vi "Data_filtering_test.vi"() -> ()   [LabVIEW 2018]
uses:
  <vilib>/Analysis/NI_AALBase.lvlib
  Tracker.lvlib
  <vilib>/Analysis/NI_AALPro.lvlib
  <vilib>/Analysis/baseanly.llb/Mean (DBL).vi
  SubVi's/Controls/CTL_Filter_selector.ctl
panel:
  out "X MSE, filt end HB":dbl format="%0.2f"
  out "Mean, coords HB + speed SG d1":dbl format="%0.2f"
  out "Speed MSE, coords HB + speed SG d1":dbl format="%0.2f"
  in  "HB filter length":i32=31
  out "Mean, coords SG + speed SG d1":dbl format="%0.2f"
  out "Mean, speed SG d1":dbl format="%0.2f"
  out "Mean, coords SG + speed HB":dbl format="%0.2f"
  out "Mean ideal speed":dbl format="%0.2f"
  out "Speed MSE, coords SG + speed HB":dbl format="%0.2f"
  out "Speed MSE, speed SG d1":dbl format="%0.2f"
  out "Speed MSE, coords SG + speed SG d1":dbl format="%0.2f"
  in  "Noise SD":dbl=3.0 min=0.0 max=10.0 step=0.1 format="%#_13g"
  out "Y MSE, filt on raw":dbl format="%0.2f"
  out "Y MSE, filt on end":dbl format="%0.2f"
  out "X MSE, filt on end":dbl format="%0.2f"
  out "X MSE, filt on raw":dbl format="%0.2f"
  out "Speed data":dbl[][](graph)
  in  "Filter parameters 2":T1={"Filter type"=enum."Savitzky-Golay", "Length"=31, "Order"=3} {"Order" min=3 max=11 step=2; "Length" min=5 max=301 step=2}
  out "Proc data":dbl[][](graph)
  in  "Filter parameters":T1={"Filter type"=enum."Savitzky-Golay", "Length"=31, "Order"=3} {"Order" min=3 max=11 step=2; "Length" min=5 max=301 step=2}
  out "Noisy raw data":dbl[][](graph)
  out "Pure raw data":dbl[][](graph)
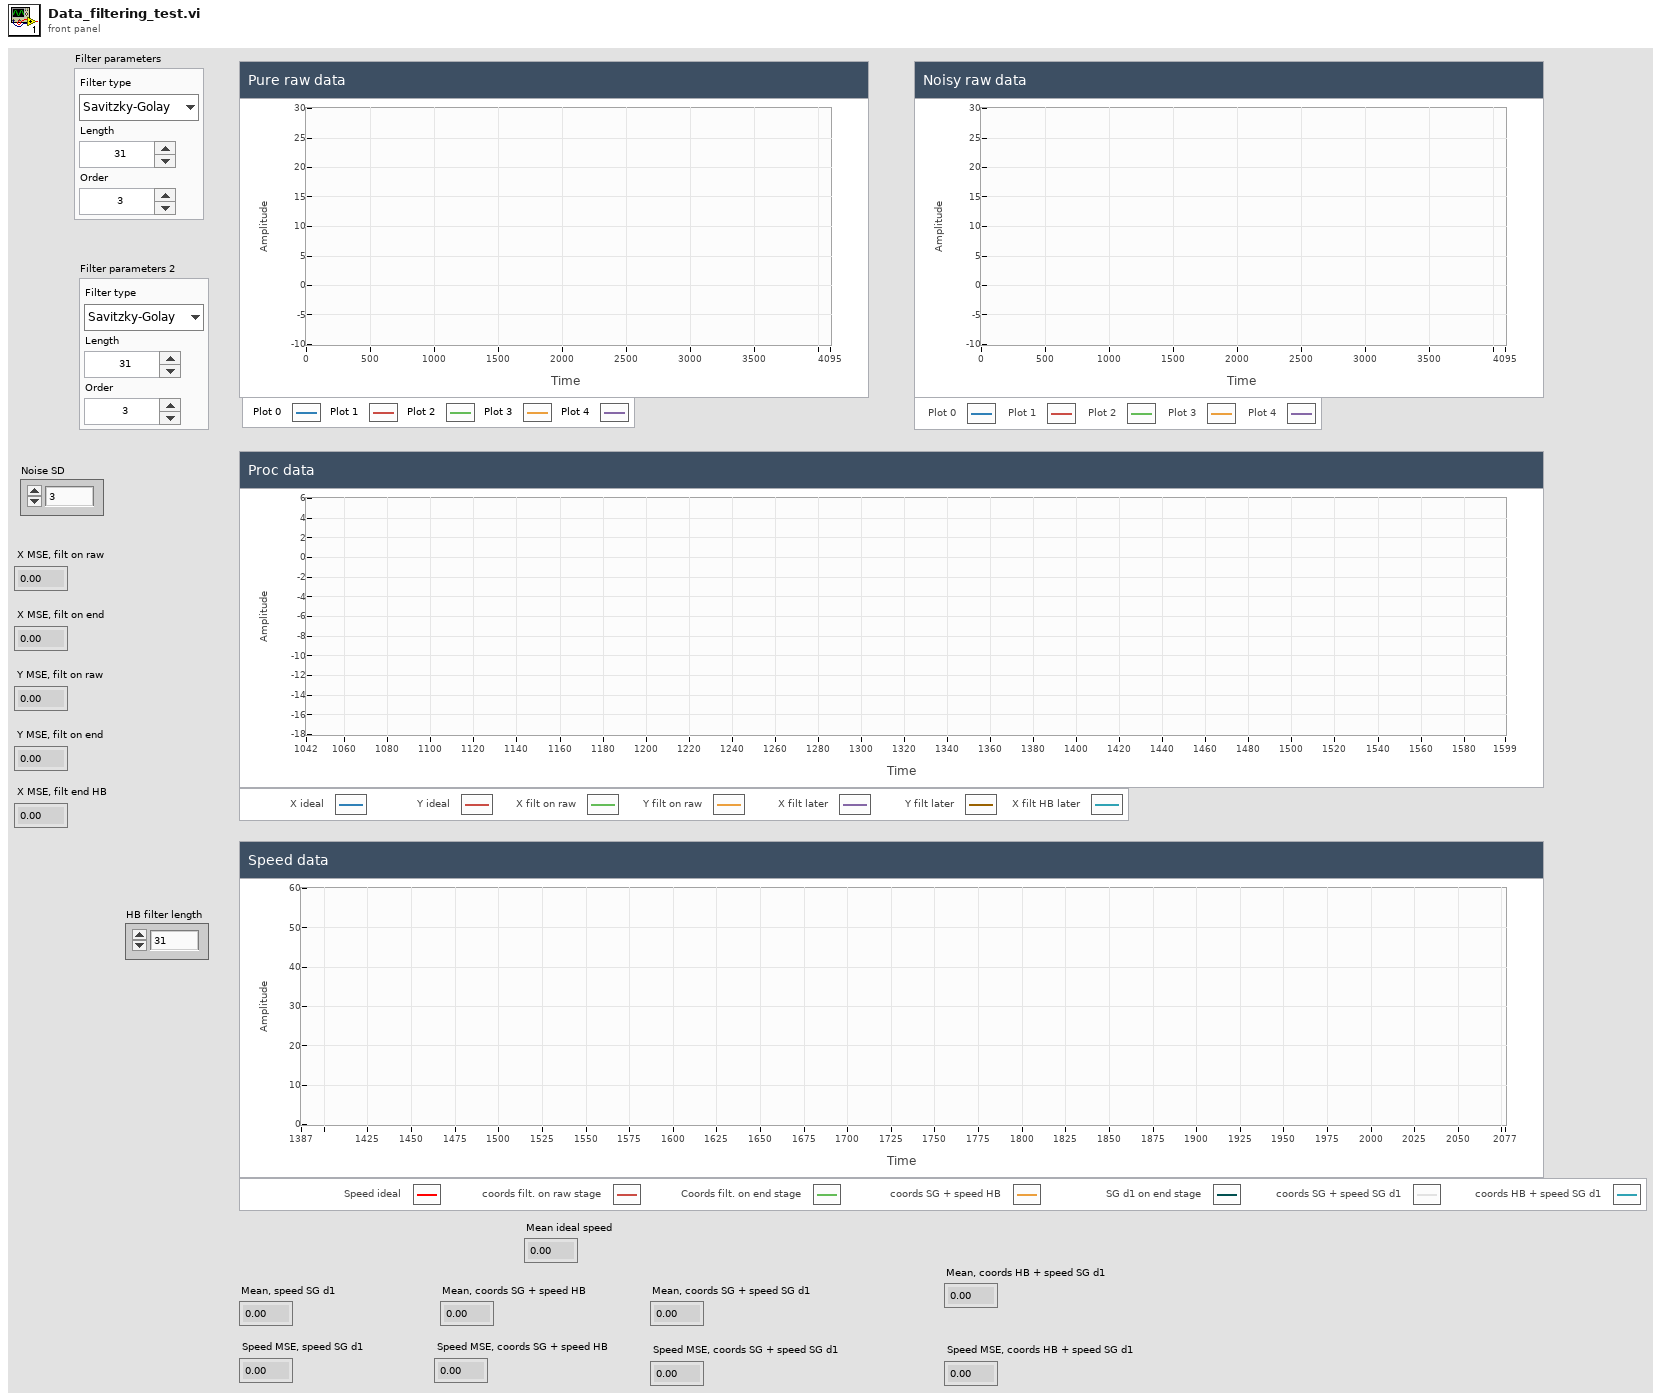
[diagram p1: front panel]
types:
  T1 = typedef "Tracker.lvlib/CTL_Filter_selector.ctl" = cluster{"Filter type":enum16{"None", "Savitzky-Golay"}, "Length":i32, "Order":i32}
  T2 = cluster{"ms since ON":u32, "delta time":u32, "X1":sgl, "Y1":sgl, "X2":sgl, "Y2":sgl, "TTL in 1":i16, "TTL in 2":i16, "Frame timestamp":timestamp, "Frame OK":bool}
  T3 = cluster{"X1 raw":dbl, "Y1 raw":dbl, "X2 raw":dbl, "Y2 raw":dbl}
  T4 = typedef "Tracker.lvlib/CTL_Cage_Coords.ctl" = cluster{"R from center":dbl, "sin(a)":dbl, "Mouse Xc":dbl, "Mouse Yc":dbl, "X1-X2":dbl, "Y1-Y2":dbl, "Cage Xc":dbl, "Cage Yc":dbl, "Frame time, s":dbl}
  T5 = cluster{"R from center":dbl, "phi (mouse angular position in the cage)":dbl, "alpha (mouse rot. angle)":sgl, "X":dbl, "Y":dbl, "theta (from center towards mouse)":dbl, "beta (cage rot. against mouse)":sgl, "w (mouse angle to wall)":dbl}
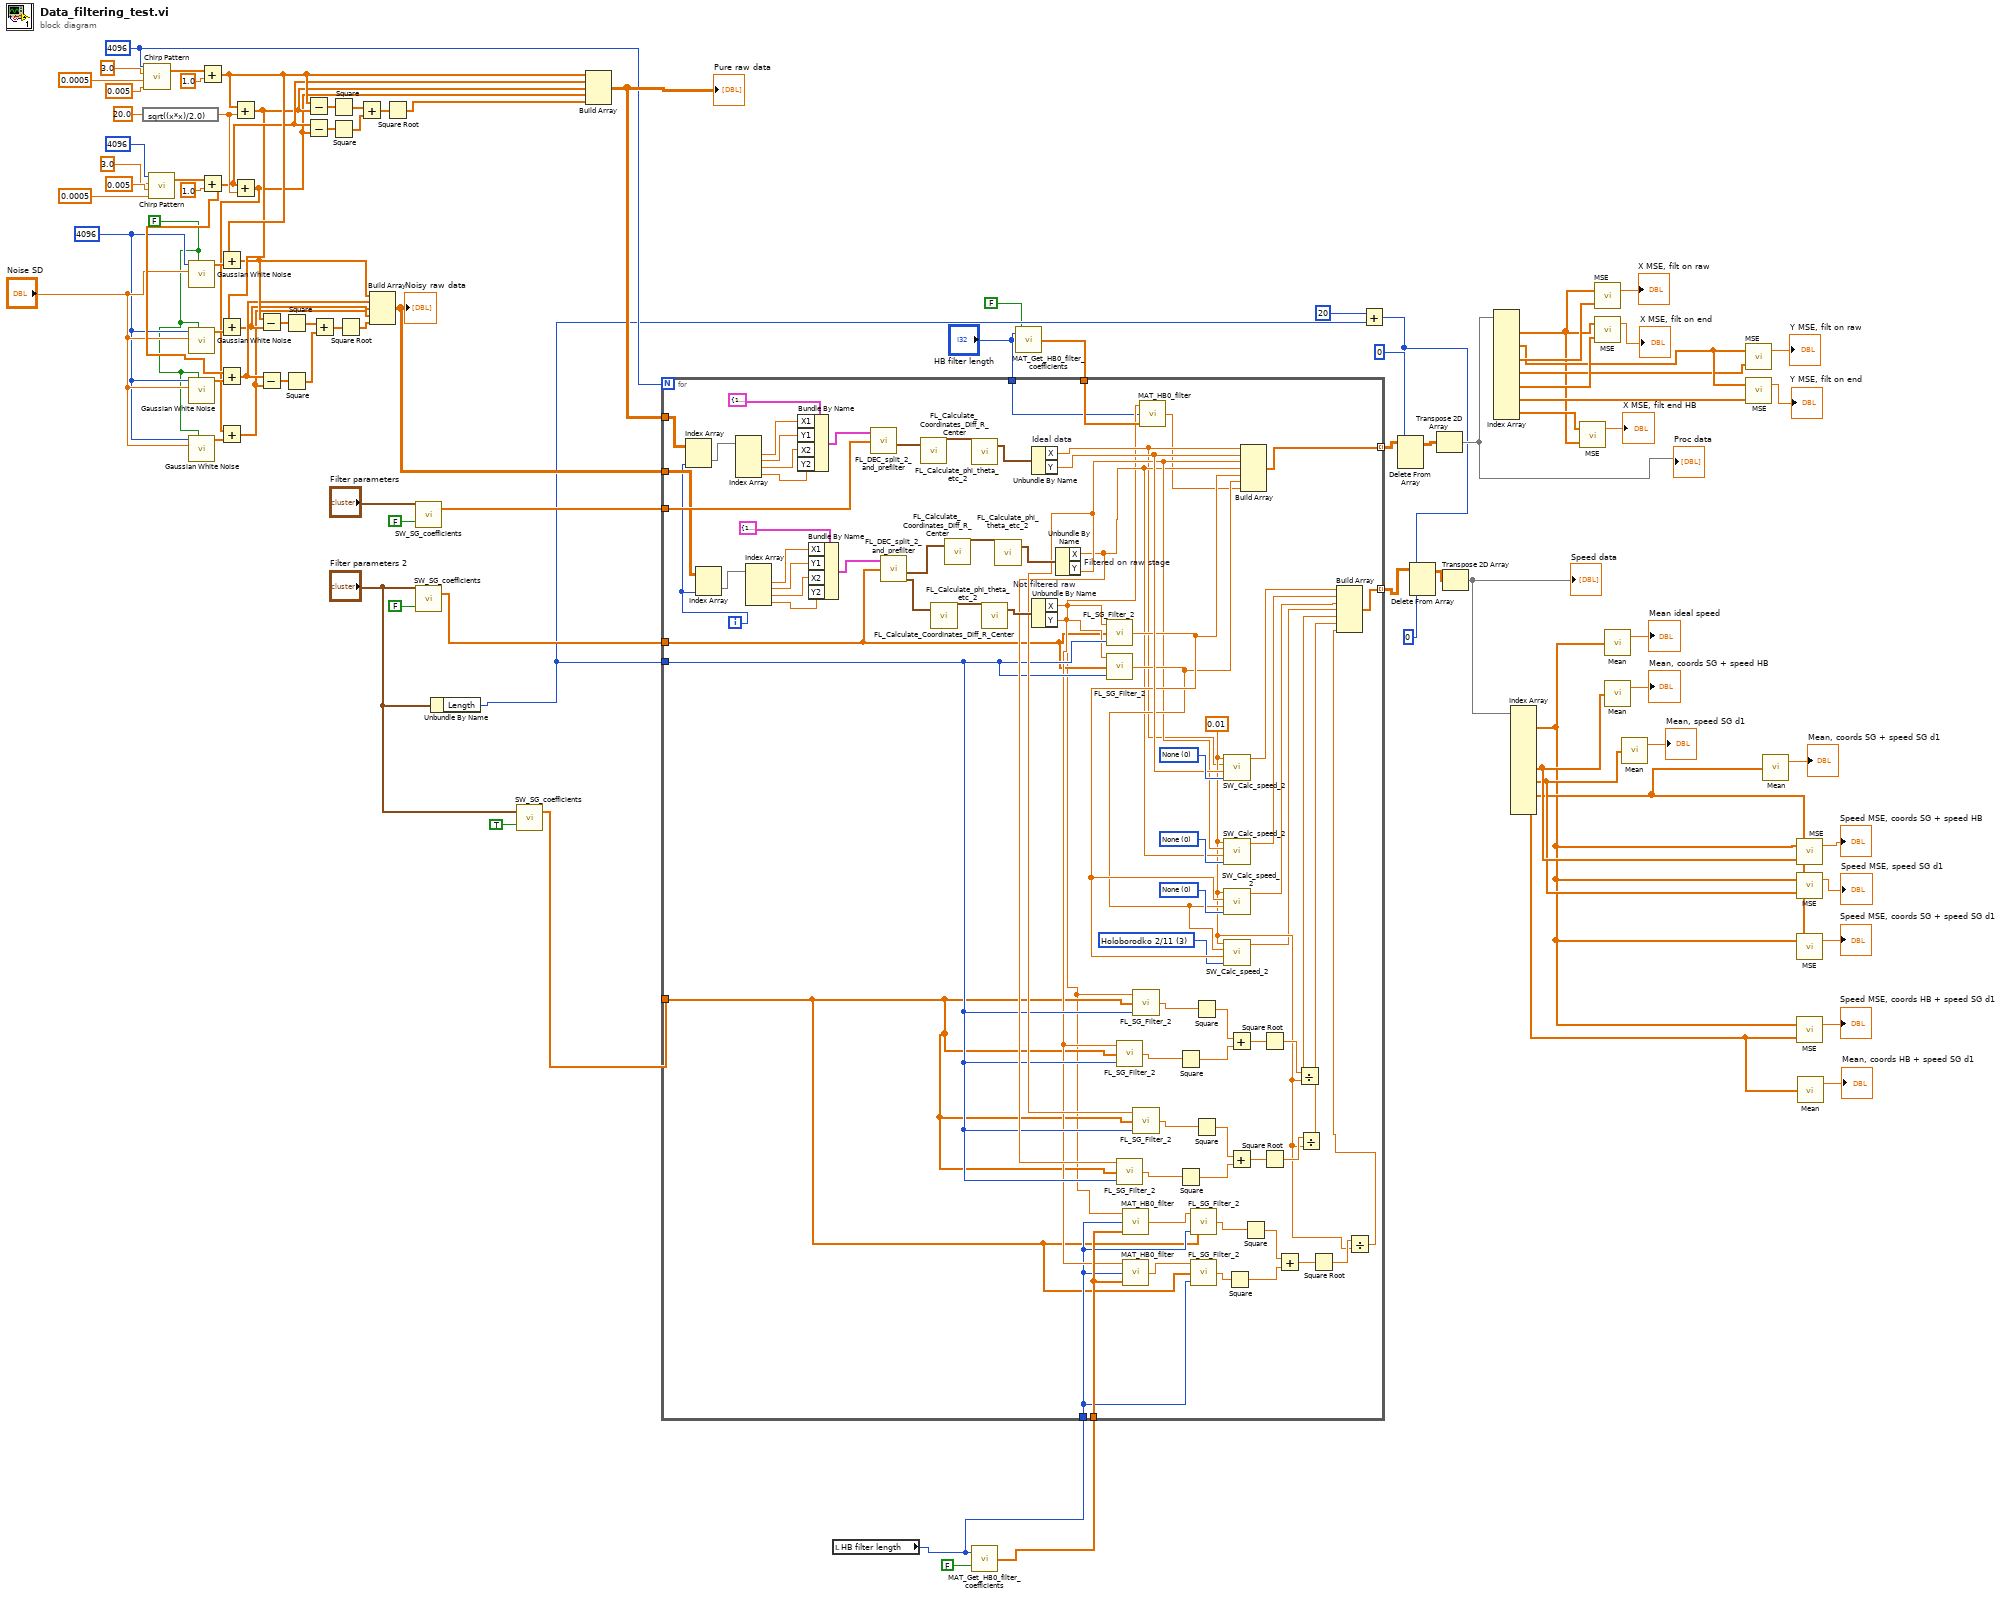
[diagram p0: block diagram]
diagram:
  w46 = FALSE ("initialize?")
  w47 = 4096 ("samples")
  w53 = 4096 ("samples")
  n1 = expression code="sqrt((x*x)/2.0)"(20.0) -> (w82:dbl)
  n2 = call <vilib>:"Chirp Pattern.vi"("f2"=0.005, "f1"=0.0005, "amplitude"=3.0, "samples"=w53) -> ("Chirp Pattern"=w91:dbl[])  [unwired: 1 out]
  n3 = call <vilib>:"Chirp Pattern.vi"("f2"=0.0005, "f1"=0.005, "amplitude"=3.0, "samples"=4096) -> ("Chirp Pattern"=w88:dbl[])  [unwired: 1 out]
  n4 = call <vilib>:"Gaussian White Noise.vi"("initialize?"=w46, "standard deviation"="Noise SD", "samples"=w47) -> ("Gaussian noise pattern"=w74:dbl[])  [unwired: 7 in, 1 out]
  n5 = call <vilib>:"Gaussian White Noise.vi"("initialize?"=w46, "standard deviation"="Noise SD", "samples"=w47) -> ("Gaussian noise pattern"=w71:dbl[])  [unwired: 7 in, 1 out]
  n6 = call <vilib>:"Gaussian White Noise.vi"("initialize?"=w46, "standard deviation"="Noise SD", "samples"=w47) -> ("Gaussian noise pattern"=w72:dbl[])  [unwired: 7 in, 1 out]
  n7 = call <vilib>:"Gaussian White Noise.vi"("initialize?"=w46, "standard deviation"="Noise SD", "samples"=w47) -> ("Gaussian noise pattern"=w68:dbl[])  [unwired: 7 in, 1 out]
  n8 = Add(x=w91, y=1.0 ("f2")) -> (x+y=w75:dbl[])
  n9 = Add(x=w88, y=1.0 ("f2")) -> (x+y=w73:dbl[])
  n10 = Add(x=w75, y=w74) -> (x+y=w62:dbl[])
  n11 = Add(x=w73, y=w72) -> (x+y=w61:dbl[])
  n12 = Add(x=w75, y=w82) -> (x+y=w70:dbl[])
  n13 = Add(x=w70, y=w71) -> (x+y=w60:dbl[])
  n14 = Add(x=w73, y=w82) -> (x+y=w69:dbl[])
  n15 = Add(x=w69, y=w68) -> (x+y=w59:dbl[])
  n16 = Subtract(x=w62, y=w60) -> (x-y=w63:dbl[])
  n17 = Subtract(x=w61, y=w59) -> (x-y=w64:dbl[])
  n18 = Square(x=w63) -> (x^2=w65:dbl[])
  n19 = Square(x=w64) -> (x^2=w66:dbl[])
  n20 = Subtract(x=w75, y=w70) -> (x-y=w81:dbl[])
  n21 = Subtract(x=w73, y=w69) -> (x-y=w80:dbl[])
  n22 = Add(x=w65, y=w66) -> (x+y=w67:dbl[])
  n23 = Square(x=w81) -> (x^2=w79:dbl[])
  n24 = Square(x=w80) -> (x^2=w78:dbl[])
  n25 = Square Root(x=w67) -> (sqrt(x)=w58:dbl[])
  n26 = Add(x=w79, y=w78) -> (x+y=w77:dbl[])
  n27 = Build Array(w62, w61, w60, w59, w58) -> (w52:dbl[][])
  "Noisy raw data" <- w52
  n28 = Square Root(x=w77) -> (sqrt(x)=w76:dbl[])
  n29 = call "SW_SG_coefficients.vi"("1st order derivative? (F)"=FALSE, "Filter parameters"="Filter parameters") -> ("SG filter coefficients"=w54:dbl[])  [unwired: 1 in]
  n30 = call "SW_SG_coefficients.vi"("1st order derivative? (F)"=FALSE, "Filter parameters"="Filter parameters 2") -> ("SG filter coefficients"=w49:dbl[])  [unwired: 1 in]
  n31 = Unbundle By Name("Filter parameters 2") -> ("Length"=w28:i32)
  n32 = call "SW_SG_coefficients.vi"("1st order derivative? (F)"=TRUE, "Filter parameters"="Filter parameters 2") -> ("SG filter coefficients"=w30:dbl[])  [unwired: 1 in]
  n33 = Build Array(w75, w73, w70, w69, w76) -> (w55:dbl[][])
  "Pure raw data" <- w55
  n34 = local read "HB filter length"() -> (w11:i32)
  n35 = call "MAT_Get_HB0_filter_coefficients.vi"("1st order derivative? (F)"=FALSE, "N"=w11) -> ("HB smoothing filter coefficients (exact up to x^4)"=w16:dbl[])
  n36 = call "MAT_Get_HB0_filter_coefficients.vi"("1st order derivative? (F)"=FALSE, "N"="HB filter length") -> ("HB smoothing filter coefficients (exact up to x^4)"=w13:dbl[])
  n37 = for {
    N: w53 -> [_]
    tunnel: w55 -> [w163]
    tunnel: w54 -> [w151]
    tunnel: [w143] -> w50 mode=indexing
    tunnel: w52 -> [w150]
    tunnel: w49 -> [w116]
    tunnel: [w140] -> w15 mode=indexing
    tunnel: w30 -> [w108]
    tunnel: w28 -> [w124]
    tunnel: w16 -> [w121]
    tunnel: w11 -> [w117]
    tunnel: w13 -> [w99]
    tunnel: "HB filter length" -> [w97]
    i -> [w149]
    w95 = u16 3 items=["None", "Holoborodko 2/5", "Holoborodko 2/7", "Holoborodko 2/11", "Holoborodko 4/7"] ("Speed smoothing type")
    w139 = u16 0 items=["None", "Holoborodko 2/5", "Holoborodko 2/7", "Holoborodko 2/11", "Holoborodko 4/7"] ("Speed smoothing type")
    w141 = u16 0 items=["None", "Holoborodko 2/5", "Holoborodko 2/7", "Holoborodko 2/11", "Holoborodko 4/7"] ("Speed smoothing type")
    w147 = u16 0 items=["None", "Holoborodko 2/5", "Holoborodko 2/7", "Holoborodko 2/11", "Holoborodko 4/7"] ("Speed smoothing type")
    w109 = 0.01 ("Time per frame, s")
    n38 = Index Array(array=w163, index (col)=w149) -> (element=w162:dbl[])  [unwired: 1 in]
    n39 = Index Array(array=w150, index (col)=w149) -> (element=w161:dbl[])  [unwired: 1 in]
    n40 = Index Array(array=w162) -> (element #1=w170:dbl, element #2=w169:dbl, element #3=w168:dbl, element #4=w148:dbl)  [unwired: 4 in]
    n41 = Index Array(array=w161) -> (element #1=w153:dbl, element #2=w154:dbl, element #3=w155:dbl, element #4=w156:dbl)  [unwired: 4 in]
    n42 = Bundle By Name(cluster=T2 {"ms since ON"=19800878, "delta time"=13, "X1"=15.131577, "Y1"=50.0, "X2"=12.5, "Y2"=-56.13208, "TTL in 1"=0, "TTL in 2"=0, "Frame timestamp"=timestamp(3638355525.2114863 s since 1904-01-01), "Frame OK"=TRUE} ("DEC input cluster"), "X1"=w170, "Y1"=w169, "X2"=w168, "Y2"=w148) -> (w167:T2)
    n43 = Bundle By Name(cluster=T2 {"ms since ON"=19800878, "delta time"=13, "X1"=15.131577, "Y1"=50.0, "X2"=12.5, "Y2"=-56.13208, "TTL in 1"=0, "TTL in 2"=0, "Frame timestamp"=timestamp(3638355525.2114863 s since 1904-01-01), "Frame OK"=TRUE} ("DEC input cluster"), "X1"=w153, "Y1"=w154, "X2"=w155, "Y2"=w156) -> (w157:T2)
    n44 = call "FL_DEC_split_2_and_prefilter.vi"("DEC input cluster"=w167, "SG filter coefficients"=w151) -> ("Magnets coords"=w166:cluster{"X1":dbl, "Y1":dbl, "X2":dbl, "Y2":dbl})  [unwired: 1 in, 3 out]
    n45 = call "FL_DEC_split_2_and_prefilter.vi"("DEC input cluster"=w157, "SG filter coefficients"=w116) -> ("Magnets coords"=w158:cluster{"X1":dbl, "Y1":dbl, "X2":dbl, "Y2":dbl}, "Magnets coords raw"=w145:T3)  [unwired: 1 in, 2 out]
    n46 = call "FL_Calculate_Coordinates_Diff_R_Center.vi"("Magnets coords in"=w166) -> ("Output cluster of data"=w165:T4)  [unwired: 2 in]
    n47 = call "FL_Calculate_Coordinates_Diff_R_Center.vi"("Magnets coords in"=w145) -> ("Output cluster of data"=w146:T4)  [unwired: 2 in]
    n48 = call "FL_Calculate_Coordinates_Diff_R_Center.vi"("Magnets coords in"=w158) -> ("Output cluster of data"=w159:T4)  [unwired: 2 in]
    n49 = call "FL_Calculate_phi_theta_etc_2.vi"("Input cluster of data"=w165) -> ("Animal coordinates"=w164:T5)  [unwired: 5 in]
    n50 = call "FL_Calculate_phi_theta_etc_2.vi"("Input cluster of data"=w146) -> ("Animal coordinates"=w144:T5)  [unwired: 5 in]
    n51 = call "FL_Calculate_phi_theta_etc_2.vi"("Input cluster of data"=w159) -> ("Animal coordinates"=w160:T5)  [unwired: 5 in]
    n52 = Unbundle By Name "Ideal data"(w164) -> ("X"=w106:dbl, "Y"=w142:dbl)
    n53 = Unbundle By Name "Not filtered raw"(w144) -> ("X"=w98:dbl, "Y"=w120:dbl)
    n54 = Unbundle By Name "Filtered on raw stage"(w160) -> ("X"=w126:dbl, "Y"=w125:dbl)
    n55 = call "FL_SG_Filter_2.vi"("N samples"=w124, "SG coefficients"=w116, "Input sample"=w98) -> ("Filtered sample"=w138:dbl)
    n56 = call "FL_SG_Filter_2.vi"("N samples"=w124, "SG coefficients"=w116, "Input sample"=w120) -> ("Filtered sample"=w137:dbl)
    n57 = call "FL_SG_Filter_2.vi"("N samples"=w124, "SG coefficients"=w108, "Input sample"=w120) -> ("Filtered sample"=w135:dbl)
    n58 = call "FL_SG_Filter_2.vi"("N samples"=w124, "SG coefficients"=w108, "Input sample"=w125) -> ("Filtered sample"=w128:dbl)
    n59 = call "MAT_HB0_filter.vi"("HB smoothing filter coefficients (exact up to x^4)"=w121, "N samples"=w117, "Input sample"=w98) -> ("Filtered sample"=w118:dbl)
    n60 = call "MAT_HB0_filter.vi"("HB smoothing filter coefficients (exact up to x^4)"=w121, "N samples"=w117, "Input sample"=w120) -> ("Filtered sample"=w119:dbl)
    n61 = call "FL_SG_Filter_2.vi"("N samples"=w124, "SG coefficients"=w108, "Input sample"=w98) -> ("Filtered sample"=w136:dbl)
    n62 = call "FL_SG_Filter_2.vi"("N samples"=w124, "SG coefficients"=w108, "Input sample"=w126) -> ("Filtered sample"=w127:dbl)
    n63 = call "MAT_HB0_filter.vi"("HB smoothing filter coefficients (exact up to x^4)"=w99, "N samples"=w97, "Input sample"=w98) -> ("Filtered sample"=w96:dbl)
    n64 = Square(x=w135) -> (x^2=w133:dbl)
    n65 = Square(x=w128) -> (x^2=w130:dbl)
    n66 = call "FL_SG_Filter_2.vi"("N samples"=w117, "SG coefficients"=w108, "Input sample"=w118) -> ("Filtered sample"=w111:dbl)
    n67 = call "FL_SG_Filter_2.vi"("N samples"=w117, "SG coefficients"=w108, "Input sample"=w119) -> ("Filtered sample"=w110:dbl)
    n68 = Square(x=w136) -> (x^2=w134:dbl)
    n69 = Square(x=w127) -> (x^2=w129:dbl)
    n70 = call "SW_Calc_speed_2.vi"("Speed smoothing type"=w147, "X coord, mm"=w142, "Y coord, mm"=w106, "Time per frame, s"=w109) -> ("Mouse speed, mm/s"=w107:dbl)  [unwired: 2 in]
    n71 = call "SW_Calc_speed_2.vi"("Speed smoothing type"=w141, "X coord, mm"=w125, "Y coord, mm"=w126, "Time per frame, s"=w109) -> ("Mouse speed, mm/s"=w105:dbl)  [unwired: 2 in]
    n72 = call "SW_Calc_speed_2.vi"("Speed smoothing type"=w139, "X coord, mm"=w137, "Y coord, mm"=w138, "Time per frame, s"=w109) -> ("Mouse speed, mm/s"=w104:dbl)  [unwired: 2 in]
    n73 = call "SW_Calc_speed_2.vi"("Speed smoothing type"=w95, "X coord, mm"=w138, "Y coord, mm"=w137, "Time per frame, s"=w109) -> ("Mouse speed, mm/s"=w103:dbl)  [unwired: 2 in]
    n74 = Square(x=w110) -> (x^2=w113:dbl)
    n75 = Add(x=w134, y=w133) -> (x+y=w132:dbl)
    n76 = Add(x=w129, y=w130) -> (x+y=w131:dbl)
    n77 = Build Array(w106, w142, w126, w125, w138, w137, w96) -> (w143:dbl[])
    n78 = Square(x=w111) -> (x^2=w114:dbl)
    n79 = Square Root(x=w132) -> (sqrt(x)=w122:dbl)
    n80 = Square Root(x=w131) -> (sqrt(x)=w123:dbl)
    n81 = Add(x=w114, y=w113) -> (x+y=w112:dbl)
    n82 = Divide(x=w122, y=w109) -> (x/y=w102:dbl)
    n83 = Divide(x=w123, y=w109) -> (x/y=w101:dbl)
    n84 = Square Root(x=w112) -> (sqrt(x)=w115:dbl)
    n85 = Divide(x=w115, y=w109) -> (x/y=w100:dbl)
    n86 = Build Array(w107, w105, w104, w103, w102, w101, w100) -> (w140:dbl[])
  }
  n87 = Add(x=20, y=w28) -> (x+y=w21:i32)
  n88 = Delete From Array(array=w50, length=w21, index (row)=0) -> (array with subset deleted=w35:dbl[][])  [unwired: 1 in, 1 out]
  n89 = Delete From Array(array=w15, length=w21, index (row)=0) -> (array with subset deleted=w32:dbl[][])  [unwired: 1 in, 1 out]
  n90 = Transpose 2D Array(2D array=w35) -> (transposed array=w36:dbl[][])
  "Proc data" <- w36
  n91 = Transpose 2D Array(2D array=w32) -> (transposed array=w14:dbl[][])
  "Speed data" <- w14
  n92 = Index Array(array=w36) -> (element #1=w4:dbl[], element #2=w39:dbl[], element #3=w45:dbl[], element #4=w38:dbl[], element #5=w44:dbl[], element #6=w37:dbl[], element #7=w5:dbl[])  [unwired: 14 in]
  n93 = Index Array(array=w14) -> (element #1=w9:dbl[], element #4=w22:dbl[], element #5=w19:dbl[], element #6=w17:dbl[], element #7=w7:dbl[])  [unwired: 14 in, 2 out]
  n94 = call <vilib>:"MSE.vi"("X Values"=w4, "Y Values"=w5) -> ("mse"=→"X MSE, filt end HB":dbl)  [unwired: 1 out]
  n95 = call <vilib>:"MSE.vi"("X Values"=w45, "Y Values"=w4) -> ("mse"=→"X MSE, filt on raw":dbl)  [unwired: 1 out]
  n96 = call <vilib>:"MSE.vi"("X Values"=w44, "Y Values"=w4) -> ("mse"=→"X MSE, filt on end":dbl)  [unwired: 1 out]
  n97 = call-poly <vilib>:"Mean.vi"("X"=w9) -> ("mean"=→"Mean ideal speed":dbl)  [unwired: 1 out]
  n98 = call-poly <vilib>:"Mean.vi"("X"=w22) -> ("mean"=→"Mean, coords SG + speed HB":dbl)  [unwired: 1 out]
  n99 = call-poly <vilib>:"Mean.vi"("X"=w19) -> ("mean"=→"Mean, speed SG d1":dbl)  [unwired: 1 out]
  n100 = call <vilib>:"MSE.vi"("X Values"=w38, "Y Values"=w39) -> ("mse"=→"Y MSE, filt on raw":dbl)  [unwired: 1 out]
  n101 = call <vilib>:"MSE.vi"("X Values"=w37, "Y Values"=w39) -> ("mse"=→"Y MSE, filt on end":dbl)  [unwired: 1 out]
  n102 = call-poly <vilib>:"Mean.vi"("X"=w17) -> ("mean"=→"Mean, coords SG + speed SG d1":dbl)  [unwired: 1 out]
  n103 = call <vilib>:"MSE.vi"("X Values"=w22, "Y Values"=w9) -> ("mse"=→"Speed MSE, coords SG + speed HB":dbl)  [unwired: 1 out]
  n104 = call <vilib>:"MSE.vi"("X Values"=w19, "Y Values"=w9) -> ("mse"=→"Speed MSE, speed SG d1":dbl)  [unwired: 1 out]
  n105 = call <vilib>:"MSE.vi"("X Values"=w17, "Y Values"=w9) -> ("mse"=→"Speed MSE, coords SG + speed SG d1":dbl)  [unwired: 1 out]
  n106 = call <vilib>:"MSE.vi"("X Values"=w7, "Y Values"=w9) -> ("mse"=→"Speed MSE, coords HB + speed SG d1":dbl)  [unwired: 1 out]
  n107 = call-poly <vilib>:"Mean.vi"("X"=w7) -> ("mean"=→"Mean, coords HB + speed SG d1":dbl)  [unwired: 1 out]
